vi "Host-Top-Level-Chirp-FFT-PowerSpectrum.vi"(8 "error in":errorcluster, 11 "Run Number\nto Load":i32=1) -> (3 "PowerSpectrum":dbl[][](array[numeric]))   [LabVIEW 2015, in "SETI_LV.lvlib"]
uses:
  SETI_LV.lvlib
  <vilib>/Analysis/2dsp.llb/Complex FFT.vi
  <vilib>/Analysis/NI_AALPro.lvlib
panel:
  in  "Max Error":dbl=0.0001 format="%#_6f"
  out "Number of Power Spectrums (from file)":i32
  out "Number of Chirp Pairs":i32
  out "Array of Greatest Error Less that 1E-5":bool[](array[boolean])
  out "Greatest Error Less that 1E-5":bool=TRUE
  out "Error (greatest to smallest)":dbl[](array[numeric]) format="%#_6f"
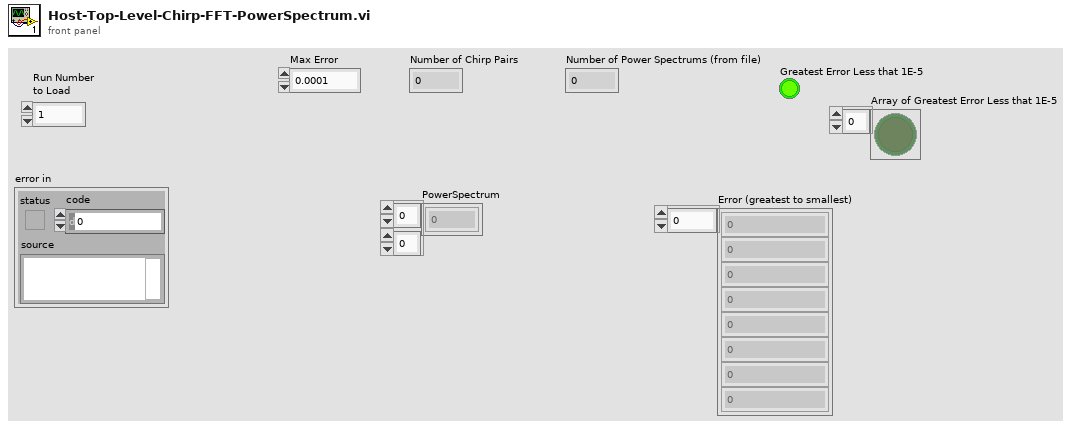
[diagram p1: front panel]
types:
  T1 = typedef "SETI_LV.lvlib/ChirpFFT Pairs.ctl" = cluster{"Chirp/Fft Pair 1 - Chirp Rate":dbl, "Chirp/Fft Pair 1 - Chirp Rate Ind":i32, "Chirp/Fft Pair 1 - Fft Length":i32, "Chirp/Fft Pair 1 - Pulse Find":i32, "Chirp/Fft Pair 1 - Gauss Fit":i32}
  T2 = typedef "SETI_LV.lvlib/Power Spectrum Data.ctl" = cluster{"icfft":i32, "NumDataPoints":i32, "Power Spectrum":sgl[]}
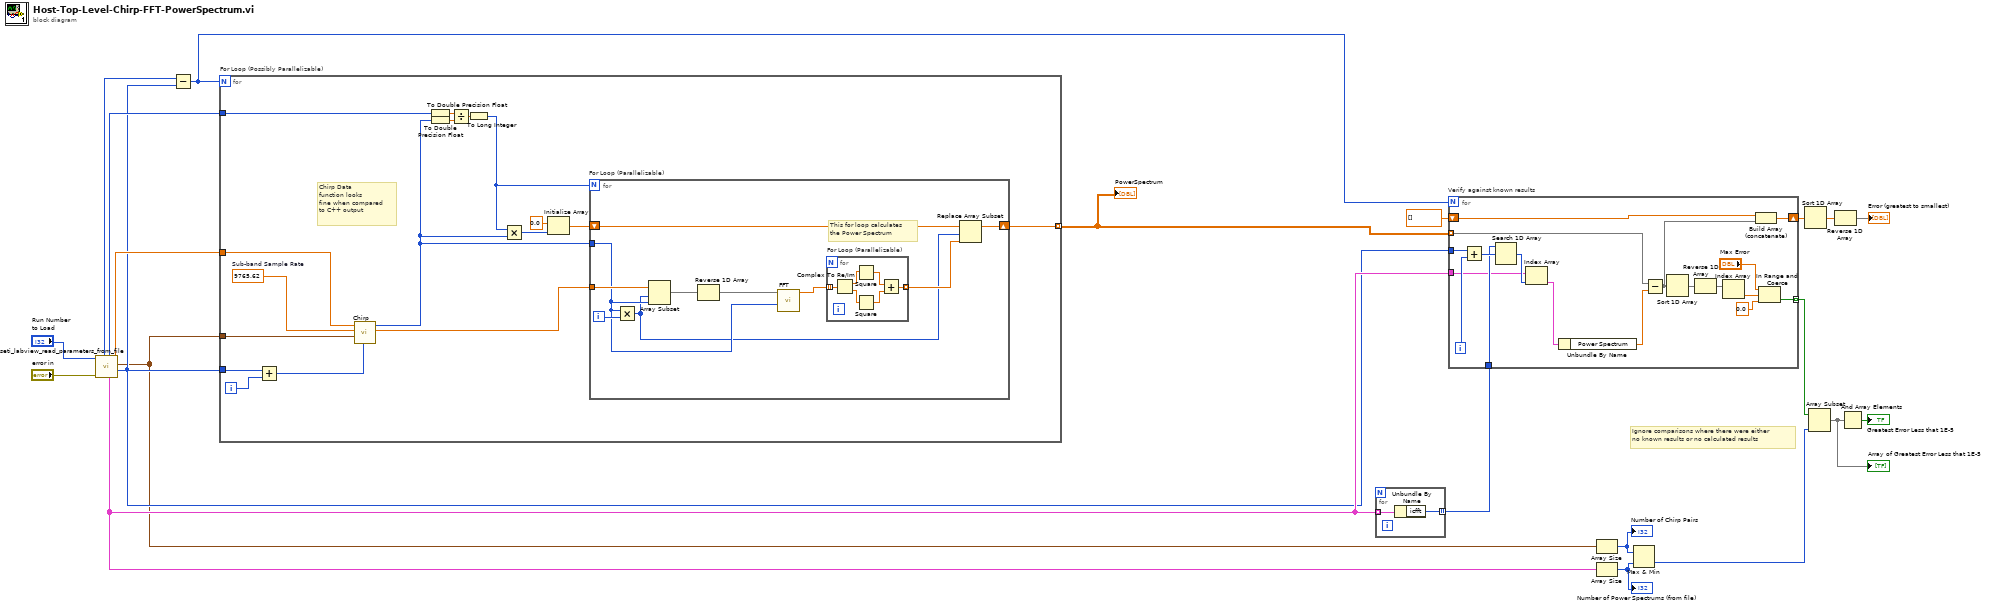
[diagram p0: block diagram]
diagram:
  # "Ignore comparisons where there were either\nno known results or no calculated results"
  n1 = call "seti_labview_read_parameters_from_file.vi"("error in (no error)"="error in", "Run Number\nto Load"="Run Number\nto Load") -> ("start_icfft"=w3:i32, "Chirp FFT Pairs"=w2:T1[], "binWorkUnitDataPoints.bin (DataIn)"=w21:csg[], "Array of Power Spectrum Data"=w9:T2[], "NumDataPoints"=w20:u32, "end_icfft"=w4:i32)  [unwired: 3 in, 1 out]
  n2 = Subtract(x=w4, y=w3) -> (x-y=w13:i32)
  n3 = for "For Loop (Possibly Parallelizable)" {
    N: w13 -> [_]
    tunnel: w3 -> [w38]
    tunnel: w2 -> [w37]
    tunnel: w21 -> [w36]
    tunnel: w20 -> [w34]
    tunnel: [w26] -> w12 mode=indexing
    i -> [w31]
    w35 = 9765.62  # Sub-band Sample Rate
    # "Chirp Data\nfunction looks\nfine when compared\nto C++ output"
    n4 = Add(x=w38, y=w31) -> (x+y=w24:i32)
    n5 = call "Chirp.vi"("icfft"=w24, "Chirp FFT Pairs"=w37, "Sub-band Sample Rate"=w35, "binWorkUnitDataPoints.bin (DataIn) in"=w36) -> ("binWorkUnitDataPoints.bin (DataIn) out"=w32:csg[], "Chirp/Fft Pair 1 - Fft Length"=w25:i32)  [unwired: 1 in, 5 out]
    n6 = To Double Precision Float(number=w34) -> (double precision float=w30:dbl)
    n7 = To Double Precision Float(number=w25) -> (double precision float=w29:dbl)
    n8 = Divide(x=w30, y=w29) -> (x/y=w33:dbl)
    n9 = To Long Integer(number=w33) -> (32bit integer=w27:i32)
    n10 = Multiply(x=w27, y=w25) -> (x*y=w22:i32)
    n11 = Initialize Array(0.0, w22) -> (w23:dbl[])
    n12 = for "For Loop (Parallelizable)" {
      N: w27 -> [_]
      tunnel: w32 -> [w48]
      tunnel: w25 -> [w43]
      shift-right: [w45] -> w26
      shift-left: w23 -> [w46]
      i -> [w47]
      # "This for loop calculates\nthe Power Spectrum"
      n13 = Multiply(x=w43, y=w47) -> (x*y=w42:i32)
      n14 = Array Subset(array=w48, index=w42, length=w43) -> (w40:csg[])
      n15 = Reverse 1D Array(array=w40) -> (reversed array=w39:csg[])
      n16 = call-poly <vilib>:"FFT.vi"("FFT size"=w43, "X"=w39) -> ("FFT {X}"=w41:cdb[])  [unwired: 8 in, 1 out]
      n17 = for "For Loop (Parallelizable)" {
        tunnel: w41 -> [w54] mode=indexing
        tunnel: [w51] -> w44 mode=indexing
        n18 = Complex To Re/Im(x + iy=w54) -> (x=w53:dbl, y=w52:dbl)
        n19 = Square(x=w53) -> (x^2=w50:dbl)
        n20 = Square(x=w52) -> (x^2=w49:dbl)
        n21 = Add(x=w50, y=w49) -> (x+y=w51:dbl)
      }
      n22 = Replace Array Subset(array=w46, new element=w44, index=w42) -> (w45:dbl[])
    }
  }
  "PowerSpectrum" <- w12
  n23 = for {
    tunnel: w9 -> [w56] mode=indexing
    tunnel: [w55] -> w11 mode=indexing
    n24 = Unbundle By Name(w56) -> ("icfft"=w55:i32)
  }
  n25 = for "Verify against known results" {
    N: w13 -> [_]
    tunnel: w12 -> [w60] mode=indexing
    tunnel: w3 -> [w73]
    tunnel: w11 -> [w70]
    tunnel: [w62] -> w10 mode=indexing
    tunnel: w9 -> [w61]
    shift-right: [w58] -> w7
    shift-left: dbl[] [] -> [w57]
    i -> [w72]
    n26 = Add(x=w73, y=w72) -> (x+y=w71:i32)
    n27 = Search 1D Array(1D array=w70, element=w71) -> (index of element=w74:i32)  [unwired: 1 in]
    n28 = Index Array(array=w61, index=w74) -> (element=w63:T2)
    n29 = Unbundle By Name(w63) -> ("Power Spectrum"=w65:sgl[])
    n30 = Subtract(x=w60, y=w65) -> (x-y=w59:dbl[])
    n31 = Sort 1D Array(array=w59) -> (sorted array=w64:dbl[])
    n32 = Reverse 1D Array(array=w64) -> (reversed array=w66:dbl[])
    n33 = Index Array(array=w66) -> (element=w69:dbl)  [unwired: 1 in]
    n34 = Build Array (concatenate)(w57, w59) -> (w58:dbl[])
    n35 = In Range and Coerce(upper limit="Max Error", x=w69, lower limit=0.0) -> (In Range?=w62:bool)  [unwired: 1 out]
  }
  n36 = Array Size(array=w2) -> (size(s)=w18:i32)
  "Number of Chirp Pairs" <- w18
  n37 = Array Size(array=w9) -> (size(s)=w15:i32)
  "Number of Power Spectrums (from file)" <- w15
  n38 = Max & Min(x=w18, y=w15) -> (min(x,y)=w16:i32)  [unwired: 1 out]
  n39 = Sort 1D Array(array=w7) -> (sorted array=w8:dbl[])
  n40 = Array Subset(array=w10, length=w16) -> (w17:bool[])  [unwired: 1 in]
  "Array of Greatest Error Less that 1E-5" <- w17
  n41 = Reverse 1D Array(array=w8) -> (reversed array=→"Error (greatest to smallest)":dbl[])
  n42 = And Array Elements(Boolean array=w17) -> (logical AND=→"Greatest Error Less that 1E-5":bool)
